vi "find_patches.vi"(5 "Shrink Factor":i32=1, 6 "Field of View":cluster{"fieldOfViewX":sgl, "fieldOfViewY":sgl}, 7 "Log File Directory":string, 8 "error in":errorcluster, 9 "debug":bool, 10 "find_patches parameters":T2, 11 "Image":T3) -> (0 "error out":errorcluster, 2 "Patches":T1(array[cluster]))   [LabVIEW 2017, in "Vision.lvlib"]
uses:
  Vision.lvlib
  <vilib>/vision/Image Controls.llb/IMAQ Image.ctl
  find_patches parameters.ctl
  bin/Vision.dll
panel:
  # "Image must be an 8-bin greyscale image"
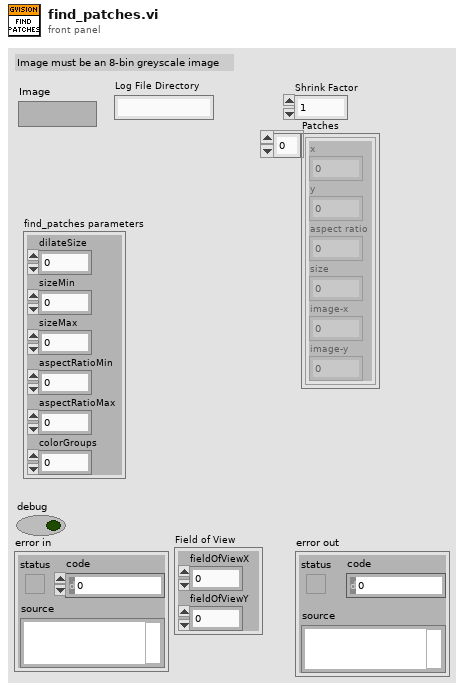
[diagram p1: front panel]
types:
  T1 = cluster{"x":dbl, "y":dbl, "aspect ratio":dbl, "size":dbl, "image-x":dbl, "image-y":dbl}[]
  T2 = typedef "Vision.lvlib/find_patches parameters.ctl" = cluster{"dilateSize":i32, "sizeMin":sgl, "sizeMax":sgl, "aspectRatioMin":sgl, "aspectRatioMax":sgl, "colorGroups":i32}
  T3 = typedef "IMAQ Image.ctl" = refnum<image>
  T4 = enum32{"Map Pixel Pointer", "Unmap Pixel Pointer", "Get Pixels Infos"}
  T5 = cluster{"x":dbl, "y":dbl, "aspect ratio":dbl, "size":dbl, "image-x":dbl, "image-y":dbl}
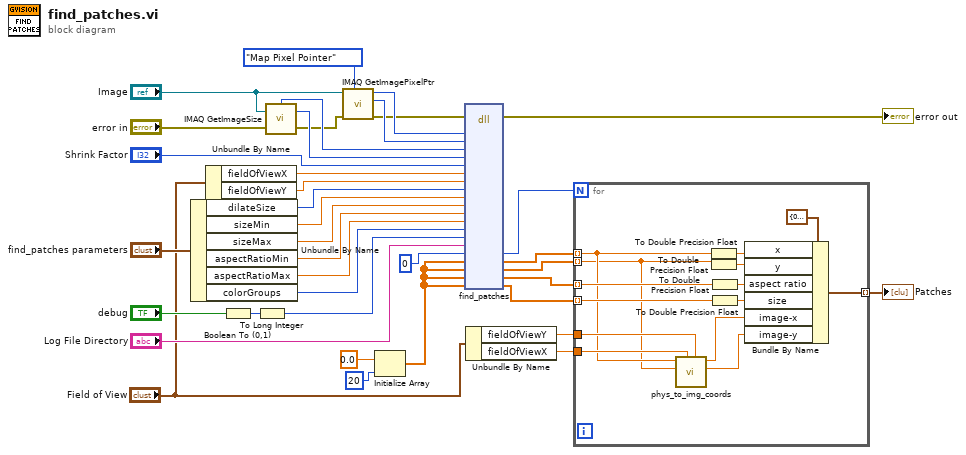
[diagram p0: block diagram]
diagram:
  n1 = Unbundle By Name("find_patches parameters") -> ("dilateSize"=w26:i32, "sizeMin"=w25:sgl, "sizeMax"=w24:sgl, "aspectRatioMin"=w23:sgl, "aspectRatioMax"=w22:sgl, "colorGroups"=w21:i32)
  n2 = Unbundle By Name("Field of View") -> ("fieldOfViewX"=w2:sgl, "fieldOfViewY"=w1:sgl)
  n3 = Boolean To (0,1)(Boolean="debug") -> (0, 1=w29:i16)
  n4 = To Long Integer(number=w29) -> (32bit integer=w28:i32)
  n5 = call "IMAQ GetImageSize"("Image"="Image", "error in (no error)"="error in") -> ("Y Resolution"=w9:i32, "X Resolution"=w10:i32, "error out"=w8:errorcluster)  [unwired: 2 in]
  n6 = call "IMAQ GetImagePixelPtr"("Function"=T4."Map Pixel Pointer", "error in (no error)"=w8, "Image"="Image") -> ("error out"=w14:errorcluster, "LineWidth(Pixels)"=w31:i32, "Pixel Pointer out"=w32:u64)  [unwired: 3 in, 3 out]
  n7 = Initialize Array(sgl 0.0 ("element"), 20 ("dimension size")) -> (w19:sgl[])
  n8 = dll-call lib="C:/Users/Caleb/Desktop/nebraska-silicon-lab/pixel-gantry-extra/LV/bin/Vision.dll" fn="find_patches"(error in=w14, "imgPtr"=w32, "imgLineWidth"=w31, "imgWidth"=w10, "imgHeight"=w9, "shrinkFactor"="Shrink Factor", "fieldOfViewX"=w2, "fieldOfViewY"=w1, "dilateSize"=w26, "sizeMin"=w25, "sizeMax"=w24, "aspectRatioMin"=w23, "aspectRatioMax"=w22, "colorGroups"=w21, "debug"=w28, "logFileDir"="Log File Directory", "numPatches"=0 ("numFiducials"), "patchXCoordinates"=w19, "patchYCoordinates"=w19, "patchAspectRatios"=w19, "patchSizes"=w19) -> (error out=→"error out":errorcluster, "numPatches"=w27:i32, "patchXCoordinates"=w18:sgl[], "patchYCoordinates"=w17:sgl[], "patchAspectRatios"=w16:sgl[], "patchSizes"=w15:sgl[])  [unwired: 18 in, 1 out]
  n9 = Unbundle By Name("Field of View") -> ("fieldOfViewY"=w6:sgl, "fieldOfViewX"=w5:sgl)
  n10 = for {
    N: w27 -> [_]
    tunnel: w18 -> [w41] mode=indexing
    tunnel: w17 -> [w40] mode=indexing
    tunnel: [w51] -> w4 mode=indexing
    tunnel: w16 -> [w46] mode=indexing
    tunnel: w15 -> [w45] mode=indexing
    tunnel: w6 -> [w43]
    tunnel: w5 -> [w42]
    n11 = call "phys_to_img_coords.vi"("fov_y"=w43, "fov_x"=w42, "y"=w40, "x"=w41) -> ("image_y"=w38:dbl, "image_x"=w39:dbl)  [unwired: 6 in]
    n12 = To Double Precision Float(number=w41) -> (double precision float=w50:dbl)
    n13 = To Double Precision Float(number=w40) -> (double precision float=w49:dbl)
    n14 = To Double Precision Float(number=w46) -> (double precision float=w48:dbl)
    n15 = To Double Precision Float(number=w45) -> (double precision float=w47:dbl)
    n16 = Bundle By Name(cluster=T5 {"x"=0.0, "y"=0.0, "aspect ratio"=0.0, "size"=0.0, "image-x"=0.0, "image-y"=0.0}, "x"=w50, "y"=w49, "aspect ratio"=w48, "size"=w47, "image-x"=w39, "image-y"=w38) -> (w51:T5)
  }
  "Patches" <- w4
